vi "channel operation tests.vi"() -> ()   [LabVIEW 2013, in "Profibus Module tests.lvlib"]
uses:
  Profibus Module tests.lvlib
  configuration/Profibus Module configuration.lvclass
panel:
  out "channels match":bool
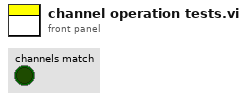
[diagram p1: front panel]
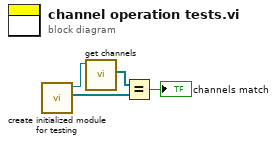
[diagram p0: block diagram]
diagram:
  n1 = call "create initialized module for testing.vi"() -> ("1d channels"=w1:refnum<class "Profibus channel.lvclass">[], "Profibus Module configuration out"=w2:refnum<class "Profibus Module configuration.lvclass">)  [unwired: 6 in, 4 out]
  n2 = call-dynamic "get channels.vi"("Profibus Module configuration in"=w2) -> ("channels"=w4:refnum<class "TBM channel.lvclass">[])  [unwired: 9 in, 1 out]
  n3 = Equal?(x=w4, y=w1) -> (x = y?=→"channels match":bool)
